vi "Main.vi"   [LabVIEW 2019]
panel:
  # "Mobile Analyzer"
types:
  T1 = typedef "AQueues.ctl" = cluster{"AccelerationRawData":refnum<queue>, "ACommand":refnum<queue>, "WebServicesAccelerationData":refnum<queue>, "AnalyzedVibrationsData":refnum<queue>}
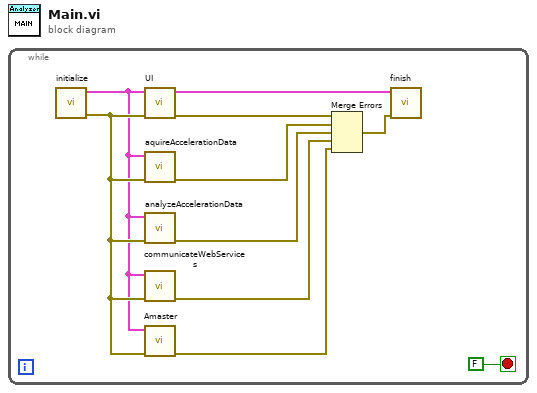
[diagram p0: block diagram]
diagram:
  n1 = while {
    stop <- FALSE stop-if-true
    n2 = call "initialize.vi"() -> ("ErrorOut"=w3:errorcluster, "Queues"=w2:T1)  [unwired: 10 in]
    n3 = call "UI.vi"("ErrorIn"=w3, "QueuesIn"=w2) -> ("ErrorOut"=w9:errorcluster, "QueuesOut"=w10:T1)  [unwired: 8 in]
    n4 = call "aquireAccelerationData.vi"("ErrorIn"=w3, "QueuesIn"=w2) -> ("ErrorOut"=w7:errorcluster)  [unwired: 8 in, 1 out]
    n5 = call "analyzeAccelerationData.vi"("ErrorIn"=w3, "QueuesIn"=w2) -> ("ErrorOut"=w8:errorcluster)  [unwired: 8 in, 1 out]
    n6 = call "communicateWebServices.vi"("ErrorIn"=w3, "QueuesIn"=w2) -> ("ErrorOut"=w5:errorcluster)  [unwired: 8 in, 1 out]
    n7 = call "Amaster.vi"("ErrorIn"=w3, "AQueuesIn"=w2) -> ("ErrorOut"=w1:errorcluster)  [unwired: 8 in, 1 out]
    n8 = Merge Errors(w9, w7, w8, w5, w1) -> (w6:errorcluster)
    n9 = call "finish.vi"("ErrorIn"=w6, "QueuesIn"=w10) -> ()  [unwired: 9 in, 1 out]
  }
